vi "create_config.vi"() -> ()   [LabVIEW 2015]
uses:
  <vilib>/Utility/config.llb/Write Key (String).vi
  <vilib>/Utility/config.llb/NI_LVConfig.lvlib
panel:
  in  "初始上传数据":string[](array[string])
  out "info_name":string[](array[string])=["用户名", "密码", "数据库名", "表名"]
  in  "info_value":string[](array[string])=["杨飞武", "898109", "yfw测试数据库", "测试13"]
  # "本模块用于手动创建配置模板"
  # "注：也可直接去网站自动生成模板"
  # "下面填入配置信息"
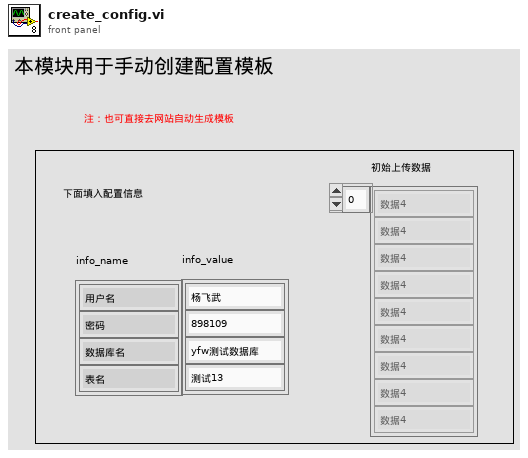
[diagram p1: front panel]
types:
  T1 = typedef "NI_LVConfig.lvlib/Config Data RefNum.ctl" = refnum<k1>
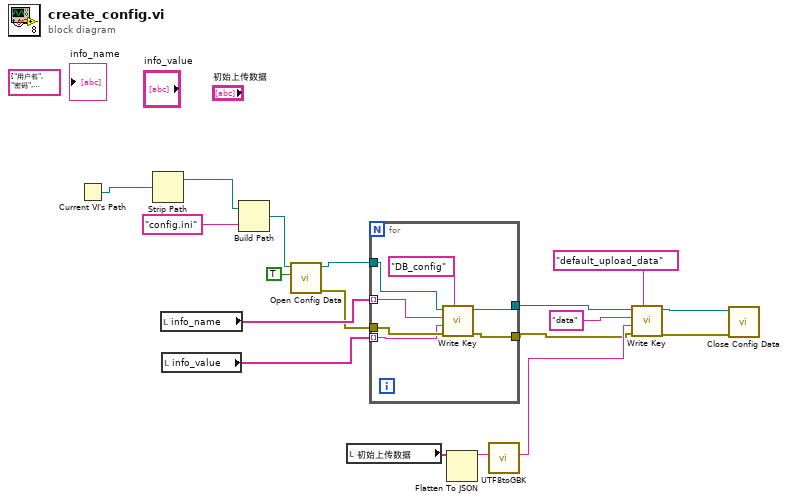
[diagram p0: block diagram]
diagram:
  (unwired) string[] ["用户名", "密码", "数据库名", "表名"] ("info_name")
  n1 = Current VI's Path() -> (path=w15:path)
  n2 = Strip Path(path=w15) -> (stripped path=w14:path)  [unwired: 1 out]
  n3 = local read "info_name"() -> (w11:string[])
  n4 = local read "info_value"() -> (w10:string[])
  n5 = Build Path(base path=w14, name or relative path="config.ini") -> (appended path=w12:path)
  n6 = call <vilib>:"Open Config Data.vi"("create file if necessary (T)"=TRUE, "configuration file path"=w12) -> ("error out"=w8:errorcluster, "refnum"=w9:T1)  [unwired: 7 in, 1 out]
  n7 = local read "初始上传数据"() -> (w18:string[])
  n8 = for {
    tunnel: w11 -> [w23] mode=indexing
    tunnel: w10 -> [w22] mode=indexing
    tunnel: w9 -> [w25]
    tunnel: w8 -> [w24]
    tunnel: [w20] -> w6
    tunnel: [w19] -> w1
    n9 = call-poly <vilib>:"Write Key.vi"("section"="DB_config", "error in (no error)"=w24, "value"=w22, "key"=w23, "refnum"=w25) -> ("error out"=w19:errorcluster, "refnum out"=w20:T1)  [unwired: 4 in, 1 out]
  }
  n10 = Flatten To JSON(anything=w18) -> (JSON string=w17:string)  [unwired: 2 in, 1 out]
  n11 = call "UTF8toGBK.vi"("UTF-8"=w17) -> ("GBK"=w4:string)  [unwired: 10 in]
  n12 = call-poly <vilib>:"Write Key.vi"("section"="default_upload_data", "error in (no error)"=w1, "value"=w4, "key"="data", "refnum"=w6) -> ("error out"=w2:errorcluster, "refnum out"=w3:T1)  [unwired: 4 in, 1 out]
  n13 = call <vilib>:"Close Config Data.vi"("error in (no error)"=w2, "refnum"=w3) -> ()  [unwired: 8 in, 2 out]
